vi "Create Channel.vi"(6 "Item Path":path, 7 "app":refnum<vi>, 11 "Element Type":variant) -> (0 "error IO":errorcluster, 3 "Channel Control Path":path)   [LabVIEW 2022 SP3, in "FlexBlocks Support.lvlib"]
uses:
  FlexBlocks Support.lvlib
  <resource>/ChannelSupport/_ChannelScriptingSupport/_ChannelScriptingSupport.lvlib
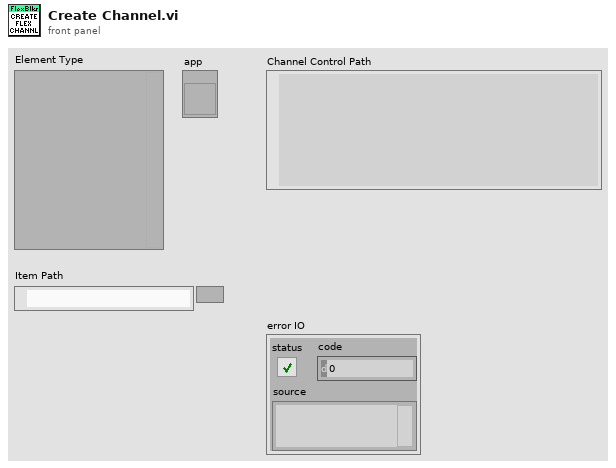
[diagram p1: front panel]
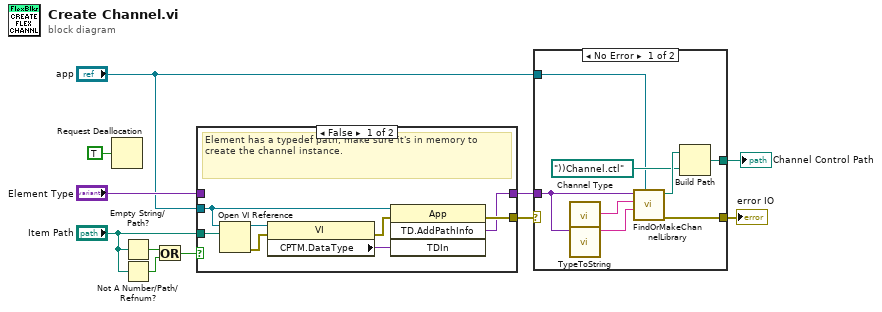
[diagram p0: block diagram]
diagram:
  n1 = Request Deallocation(TRUE ("flag")) -> ()
  n2 = Empty String/Path?(string/path="Item Path") -> (empty?=w11:bool)
  n3 = Not A Number/Path/Refnum?(number/path/refnum="Item Path") -> (NaN/Path/Refnum?=w10:bool)
  n4 = Or(x=w11, y=w10) -> (x .or. y?=w6:bool)
  n5 = case shown="False" w6 {
    tunnel: "Item Path" -> [w18 _]
    tunnel: "Element Type" -> [_ w20]
    tunnel: [w12 w20] -> w1
    tunnel: "app" -> [w15 _]
    tunnel: [w14 _] -> w7
    frame False {
      # "Element has a typedef path, make sure it's in memory to create the channel instance."
      n6 = Open VI Reference(application reference (local)=w15, vi path=w18) -> (vi reference=w17:refnum<vi>, error out=w16:errorcluster)  [unwired: 4 in]
      n7 = property class="VI"(reference=w17, error in=w16) -> (error out=w19:errorcluster, "CPTM.DataType"=w13:variant)  [unwired: 1 out]
      n8 = invoke class="App" method="TD.AddPathInfo"(reference=w15, error in=w19, "TDIn"=w13) -> (error out=w14:errorcluster, "TD.AddPathInfo"=w12:variant)  [unwired: 1 in, 2 out]
    }
    frame True {
      # "Element is not a typedef, can create channel directly from it."
    }
  }
  n9 = case shown="No Error" w7 {
    selector: w7 -> [_ w29]
    tunnel: "app" -> [w23 _]
    tunnel: w1 -> [w22 _]
    tunnel: [w24 _] -> w4
    tunnel: [w28 w29] -> w3
    frame No Error {
      n10 = call "Channel Type.vi"() -> ("Channel Template"=w21:string)  [unwired: 11 in]
      n11 = call <resource>:"TypeToString.vi"("type"=w22) -> ("string"=w27:string)  [unwired: 10 in]
      n12 = call <resource>:"FindOrMakeChannelLibrary.vi"("app"=w23, "typestring"=w27, "class"=w21, "elt type"=w22) -> ("error out"=w28:errorcluster, "channel folder"=w26:path)  [unwired: 6 in]
      n13 = Build Path(base path=w26, name or relative path=path "))Channel.ctl") -> (appended path=w24:path)
    }
    frame Error {
    }
  }
  "Channel Control Path" <- w4
  "error IO" <- w3
